vi "WriteControlWord.vi"(8 "error in (no error)":errorcluster, 10 "Controlword":string(combo), 11 "Motor Base in":refnum<class "Motor Base.lvclass">) -> (0 "error out":errorcluster, 3 "Motor Base out":refnum<class "Motor Base.lvclass">)   [LabVIEW 2016, in "Motor Base.lvlib" / "Motor Base.lvclass"]
uses:
  Motor Base.lvclass
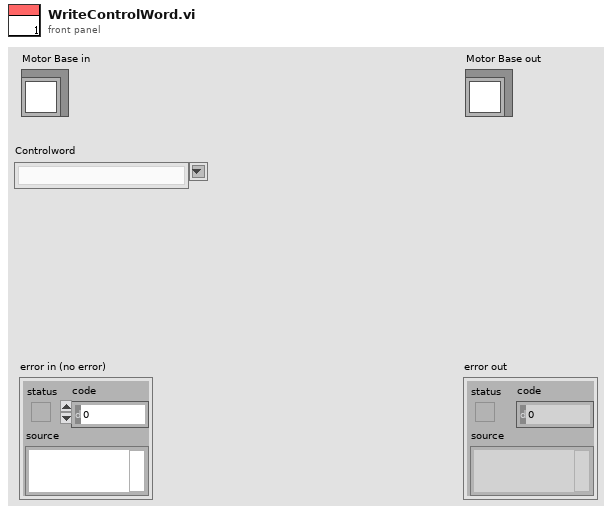
[diagram p1: front panel]
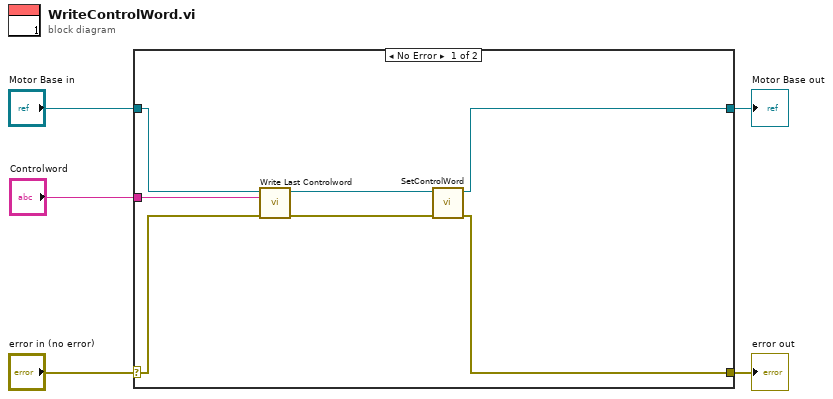
[diagram p0: block diagram]
diagram:
  n1 = case shown="No Error" "error in (no error)" {
    selector: "error in (no error)" -> [w10 w14]
    tunnel: [w6 w14] -> w4
    tunnel: [w7 w13] -> w2
    tunnel: "Motor Base in" -> [w11 w13]
    tunnel: "Controlword" -> [w12 _]
    frame No Error {
      n2 = call-dynamic "Write Last Controlword.vi"("error in (no error)"=w10, "Controlword"=w12, "Motor Base in"=w11) -> ("error out"=w8:errorcluster, "Motor Base out"=w9:refnum<class "Motor Base.lvclass">)  [unwired: 7 in]
      n3 = call-dynamic "SetControlWord.vi"("error in (no error)"=w8, "Motor Base in"=w9) -> ("error out"=w6:errorcluster, "Motor Base out"=w7:refnum<class "Motor Base.lvclass">)  [unwired: 8 in]
    }
    frame Error {
    }
  }
  "error out" <- w4
  "Motor Base out" <- w2
